vi "DAQmx Write (Analog 1D DBL 1Chan NSamp).vi"(0 "task/channels in":refnum<k21>, 1 "auto start":bool, 7 "data":dbl[](array[numeric]) format="%0.2f", 9 "timeout":dbl=10.0 format="%0.2f", 11 "error in":errorcluster) -> (4 "task out":refnum<k21>, 10 "number of samples written per channel":u32, 15 "error out":errorcluster)   [LabVIEW 2013]
doc: "Writes one or more floating-point samples to a task that contains a single analog output channel."
uses:
  nilvaiu.dll
panel:
  # "sample #"
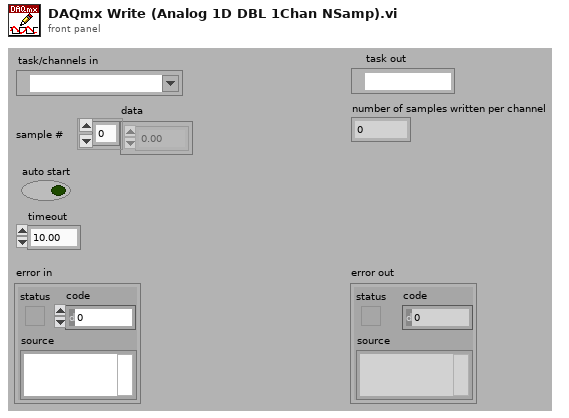
[diagram p1: front panel]
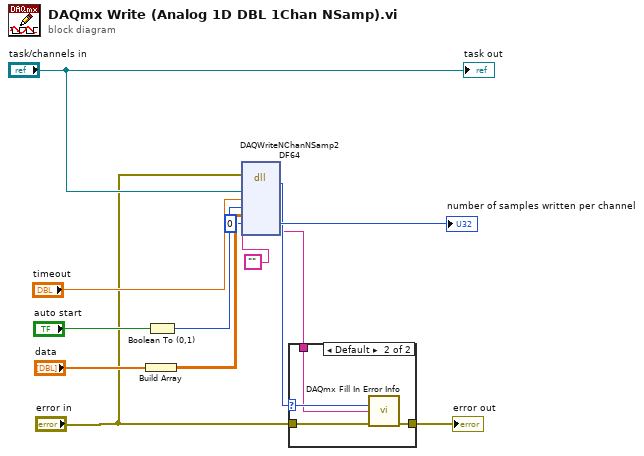
[diagram p0: block diagram]
diagram:
  n1 = Build Array("data") -> (w5:dbl[][])
  n2 = Boolean To (0,1)(Boolean="auto start") -> (0, 1=w6:i16)
  n3 = dll-call lib="nilvaiu.*" fn="DAQWriteNChanNSamp2DF64"(error in="error in", "taskID"="task/channels in", "timeout"="timeout", "autoStart"=w6, "data"=w5, "numSamplesWriten"=u32 0, "extendedErrorInfo"="") -> (w7:i32, "numSamplesWriten"=→"number of samples written per channel":u32, "extendedErrorInfo"=w3:string)  [unwired: 4 in, 4 out]
  n4 = case shown="Default" w7 {
    selector: w7 -> [_ w16]
    tunnel: "error in" -> [w14 w18]
    tunnel: [w14 w17] -> w12
    tunnel: w3 -> [_ w15]
    frame 0 {
    }
    frame Default {
      n5 = call "DAQmx Fill In Error Info.vi"("status code"=w16, "extended error info"=w15, "error in"=w18) -> ("error out"=w17:errorcluster)  [unwired: 1 in, 11 out]
    }
  }
  "error out" <- w12
  "task out" <- "task/channels in"
